vi "ConnectToSplash.vi"   [LabVIEW 2025]
uses:
  StartupSplash/StartupSplash.lvclass
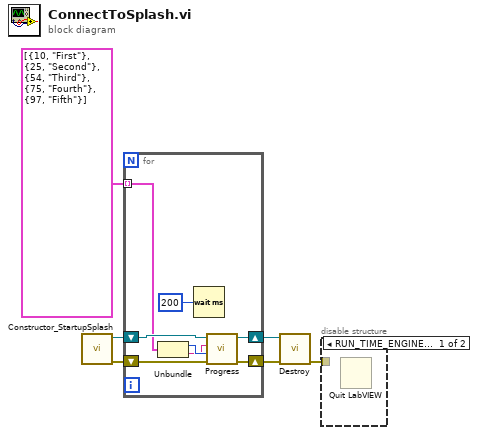
[diagram p0: block diagram]
diagram:
  n1 = call "Constructor_StartupSplash.vi"() -> ("error out"=w6:errorcluster, "StartupSplash out"=w5:refnum<class "StartupSplash.lvclass">)  [unwired: 10 in]
  n2 = for {
    shift-right: [w11] -> w3
    shift-left: w5 -> [w12]
    shift-right: [w10] -> w2
    shift-left: w6 -> [w13]
    tunnel: cluster{i32, string}[] [{10, "First"}, {25, "Second"}, {54, "Third"}, {75, "Fourth"}, {97, "Fifth"}] -> [w9] mode=indexing
    n3 = Unbundle(w9) -> (w8:i32, w7:string)
    n4 = Wait (ms)(milliseconds to wait=u32 200) -> ()  [unwired: 1 out]
    n5 = call "Progress.vi"("error in (no error)"=w13, "Progress (%)"=w8, "Message"=w7, "StartupSplash in"=w12) -> ("error out"=w10:errorcluster, "StartupSplash out"=w11:refnum<class "StartupSplash.lvclass">)  [unwired: 6 in]
  }
  n6 = call "Destroy.vi"("error in (no error)"=w2, "StartupSplash in"=w3) -> ("error out"=w1:errorcluster)  [unwired: 9 in]
  n7 = disable-structure shown="RUN_TIME_ENGINE==True" {
    disable-tunnel: w1 -> [_ _]
    frame condition #0 {
      n8 = Quit LabVIEW() -> ()  [unwired: 1 in]
    }
    frame condition #1 (active) {
    }
  }
